vi "close.vi"(8 "error in (no error)":errorcluster caption="错误输入（无错误）", 11 "2700 输入":refnum<class "2700.lvclass">) -> (0 "error out":errorcluster caption="错误输出", 3 "2700 输出":refnum<class "2700.lvclass">)   [LabVIEW 2021, in "2700.lvclass"]
uses:
  2700.lvclass
  2700.lvclass/2700.ctl
  <instrlib>/Keithley 27XX/Keithley 27XX.lvlib
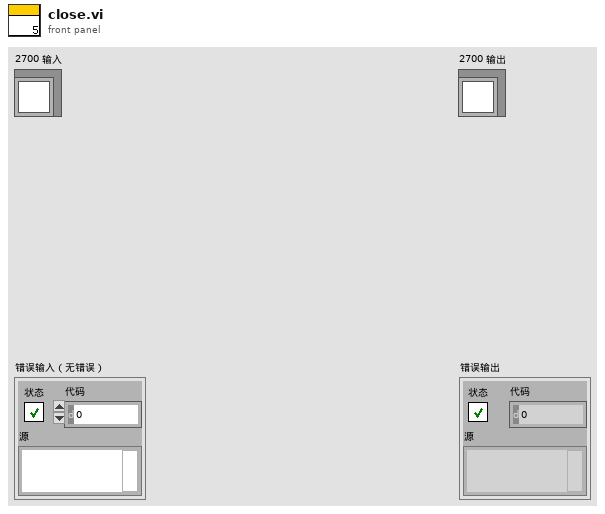
[diagram p1: front panel]
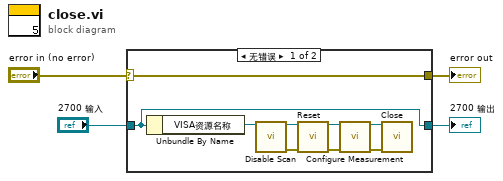
[diagram p0: block diagram]
diagram:
  n1 = case shown="无错误" "error in (no error)" {
    selector: "error in (no error)" -> [w12 w14]
    tunnel: "2700 输入" -> [w13 w15]
    tunnel: [w13 w15] -> w2
    tunnel: [w12 w14] -> w1
    frame No Error {
      n2 = Unbundle By Name(w13) -> ("VISA资源名称"=w11:refnum<visa-resource-name>)
      n3 = call <instrlib>:"Disable Scan.vi"("VISA resource name"=w11) -> ("VISA resource name out"=w9:refnum<visa-resource-name>, "error out"=w10:errorcluster)  [unwired: 13 in]
      n4 = call <instrlib>:"Reset.vi"("VISA resource name"=w9, "error in (no error)"=w10) -> ("VISA resource name out"=w8:refnum<visa-resource-name>, "error out"=w7:errorcluster)  [unwired: 12 in]
      n5 = call <instrlib>:"Configure Measurement.vi"("VISA resource name"=w8, "error in (no error)"=w7) -> ("VISA resource name out"=w6:refnum<visa-resource-name>, "error out"=w5:errorcluster)  [unwired: 12 in]
      n6 = call <instrlib>:"Close.vi"("VISA resource name"=w6, "error in (no error)"=w5) -> ()  [unwired: 13 in, 1 out]
    }
    frame Error {
    }
  }
  "error out" <- w1
  "2700 输出" <- w2
